vi "567.vi"() -> ()   [LabVIEW 2017]
uses:
  <vilib>/userdefined/High Color/IMAQdx.ctl
  <vilib>/vision/driver/NI_Vision_Acquisition_Software.lvlib
panel:
  out "Image":T1(plugin-control)
  out "X":sgl
  out "Edges Coordinates (Edge Detector 1)":cluster{"X":sgl, "Y":sgl}[](array[cluster]) {"Y" format="%.2f"; "X" format="%.2f"}
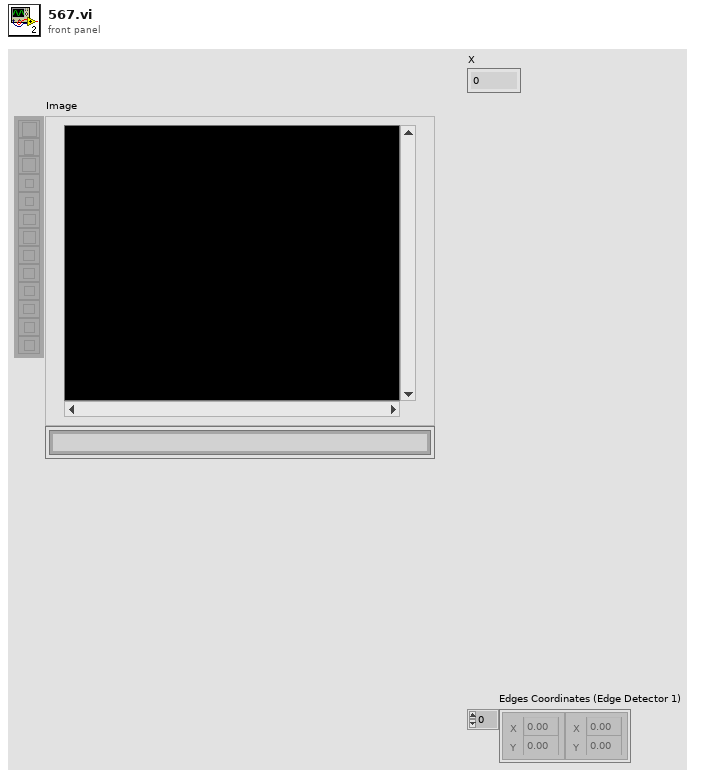
[diagram p1: front panel]
types:
  T1 = typedef "IMAQ Image.ctl" = refnum<image>
  T2 = typedef "IMAQdx.ctl" = refnum<k21>
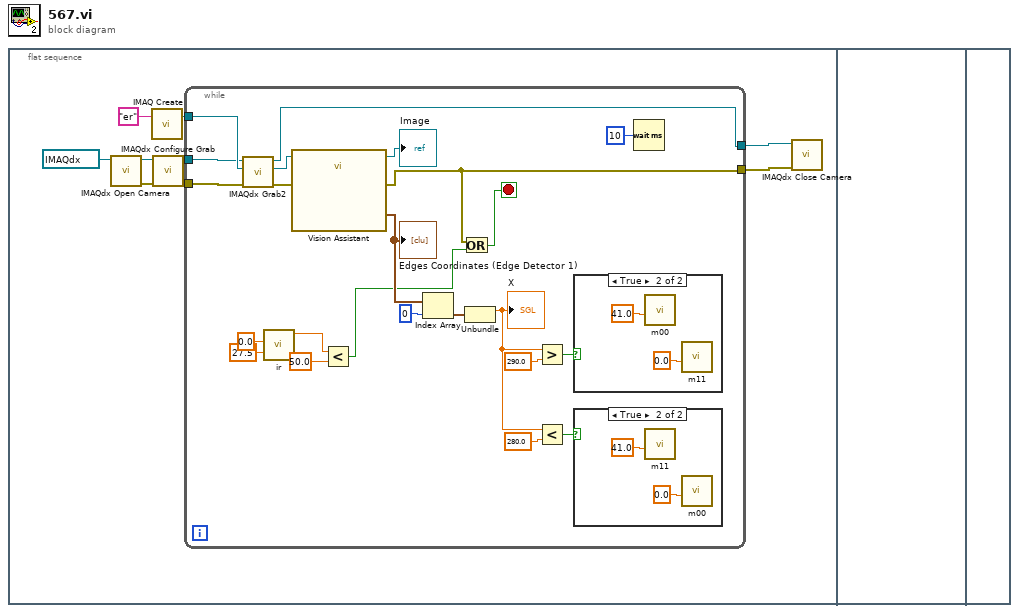
[diagram p0: block diagram]
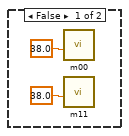
[diagram p2: hidden frame]
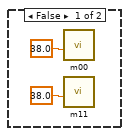
[diagram p3: hidden frame]
diagram:
  n1 = flat-sequence {
    frame #0 {
      n2 = call <vilib>:"IMAQdx Open Camera.vi"("Session In"=T2 "cam1") -> ("error out"=w6:errorcluster, "Session Out"=w5:T2)  [unwired: 9 in]
      n3 = call "IMAQ Create"("Image Name"="er") -> ("New Image"=w3:T1)  [unwired: 4 in, 1 out]
      n4 = call <vilib>:"IMAQdx Configure Grab.vi"("error in"=w6, "Session In"=w5) -> ("error out"=w7:errorcluster, "Session Out"=w4:T2)  [unwired: 8 in]
      n5 = while {
        tunnel: w7 -> [w23]
        tunnel: w3 -> [w22]
        tunnel: w4 -> [w21]
        tunnel: [w20] -> w9
        tunnel: [w16] -> w8
        stop <- w17 stop-if-true
        n6 = call <vilib>:"IMAQdx Grab2.vi"("error in"=w23, "Image In"=w22, "Session In"=w21) -> ("error out"=w26:errorcluster, "Image Out"=w25:T1, "Session Out"=w20:T2)  [unwired: 5 in, 1 out]
        n7 = call "ir.vi"("Koffset [cm]"=0.0, "Kscale [cm-V]"=27.5) -> ("см"=w14:dbl)  [unwired: 8 in, 1 out]
        n8 = call "Vision Assistant"("Image In"=w25, "error in"=w26) -> ("Image Out"=→"Image":T1, "Edges Coordinates (Edge Detector 1)"=w29:cluster{"X":sgl, "Y":sgl}[], "error out"=w16:errorcluster)  [unwired: 23 in]
        "Edges Coordinates (Edge Detector 1)" <- w29
        n9 = Less?(x=w14, y=50.0) -> (x < y?=w12:bool)
        n10 = Index Array(array=w29, index=0) -> (element=w28:cluster{"X":sgl, "Y":sgl})
        n11 = Or(x=w16, y=w12) -> (x .or. y?=w17:bool)
        n12 = Unbundle(w28) -> ("X"=w30:sgl)  [unwired: 1 out]
        "X" <- w30
        n13 = Greater?(x=w30, y=sgl 290.0) -> (0:w19:bool)
        n14 = Less?(x=w30, y=sgl 280.0) -> (x < y?=w18:bool)
        n15 = case shown="True" w19 {
          frame False {
            n16 = call "m00.vi"("position"=38.0) -> ()  [unwired: 10 in, 1 out]
            n17 = call "m11.vi"("position"=38.0) -> ()  [unwired: 10 in, 1 out]
          }
          frame True {
            n18 = call "m00.vi"("position"=41.0) -> ()  [unwired: 10 in, 1 out]
            n19 = call "m11.vi"("position"=0.0) -> ()  [unwired: 10 in, 1 out]
          }
        }
        n20 = case shown="True" w18 {
          frame False {
            n21 = call "m00.vi"("position"=38.0) -> ()  [unwired: 10 in, 1 out]
            n22 = call "m11.vi"("position"=38.0) -> ()  [unwired: 10 in, 1 out]
          }
          frame True {
            n23 = call "m11.vi"("position"=41.0) -> ()  [unwired: 10 in, 1 out]
            n24 = call "m00.vi"("position"=0.0) -> ()  [unwired: 10 in, 1 out]
          }
        }
        n25 = Wait (ms)(milliseconds to wait=u32 10) -> ()  [unwired: 1 out]
      }
      n26 = call <vilib>:"IMAQdx Close Camera.vi"("error in"=w8, "Session In"=w9) -> ()  [unwired: 9 in, 1 out]
    }
    frame #1 {
    }
    frame #2 {
    }
  }
